vi "LabVIEW Data to Python String (CSG).vi"(8 "error in (no error)":errorcluster, 10 "LabVIEW Data":csg) -> (0 "error out":errorcluster, 2 "Python String":string)   [LabVIEW 2020, in "jki_python_data_tools.lvlib"]
doc: "Writes a value associated with key in a specified section of the configuration data identified by refnum. If \"key\" input is not specified, the name of the variant object is used as the key.\n\nFor example a Boolean named \"Enable\" with a value of TRUE would correspond to the key-value pair:\n\nEnable=TRUE"
uses:
  jki_python_data_tools.lvlib
panel:
  # "Copyright © 2003-2009 JKI. All rights reserved.\n\nAuthor: Jim Kring [jim.kring@jameskring.com]\n\nThis library is provided \"AS IS\" ,WITHOUT WARRANTIES OR \nCONDITIONS OF ANY KIND, either express or implied.\n\nJames Kring, Inc. -- http://www.jameskring.com"
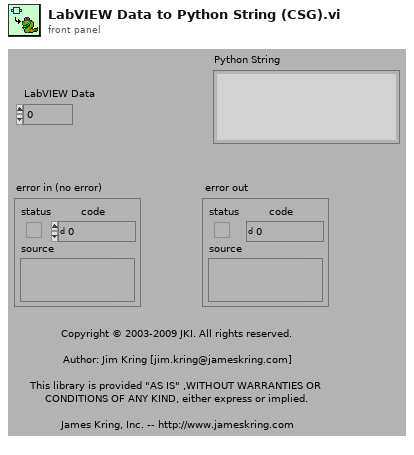
[diagram p1: front panel]
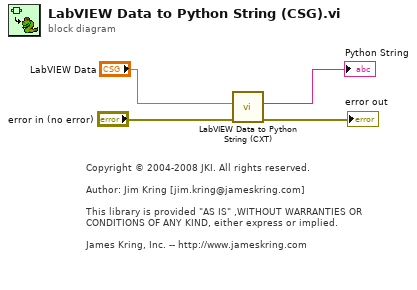
[diagram p0: block diagram]
diagram:
  # "Copyright © 2004-2008 JKI. All rights reserved.\n\nAuthor: Jim Kring [jim.kring@jameskring.com]\n\nThis library is provided \"AS IS\" ,WITHOUT WARRANTIES OR \nCONDITIONS OF ANY KIND, either express or implied.\n\nJames Kring, Inc. -- http://www.jameskring.com"
  n1 = call "LabVIEW Data to Python String (CXT).vi"("error in (no error)"="error in (no error)", "LabVIEW Data"="LabVIEW Data") -> ("error out"=→"error out":errorcluster, "Python String"=→"Python String":string)  [unwired: 8 in]
